vi "Generate Event.vi"(0 "Event":refnum<user-event>, 5 "Type":T1, 7 "New row":i32=-1, 9 "Old row":i32=-1, 11 "Data":variant) -> (4 "Event out":refnum<user-event>)   [LabVIEW 2020, in "KTable.xctl"]
uses:
  KTable.xctl
  Event Type.ctl
  Event Data.ctl
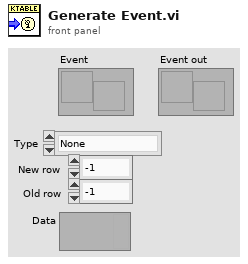
[diagram p1: front panel]
types:
  T1 = typedef "KTable.xctl/Event Type.ctl" = enum16{"None", "Selection", "Edit", "Insert", "Delete", "Up", "Down", "Duplicate"}
  T2 = typedef "KTable.xctl/Event Data.ctl" = cluster{"Type":T1, "New row":i32, "Old row":i32, "Data":variant}
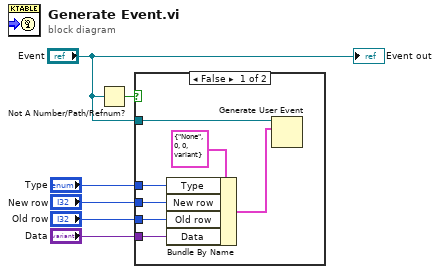
[diagram p0: block diagram]
diagram:
  n1 = Not A Number/Path/Refnum?(number/path/refnum="Event") -> (NaN/Path/Refnum?=w6:bool)
  n2 = case shown="False" w6 {
    tunnel: "Event" -> [w13 _]
    tunnel: "Type" -> [w10 _]
    tunnel: "New row" -> [w9 _]
    tunnel: "Old row" -> [w8 _]
    tunnel: "Data" -> [w7 _]
    frame False {
      n3 = Bundle By Name(cluster=T2 {"Type"=enum."None", "New row"=0, "Old row"=0, "Data"=variant} ("Event Data"), "Type"=w10, "New row"=w9, "Old row"=w8, "Data"=w7) -> (w11:T2)
      n4 = Generate User Event(user event=w13, event data cluster=w11) -> ()  [unwired: 2 in, 2 out]
    }
    frame True {
    }
  }
  "Event out" <- "Event"
